vi "DBValueToDBSignal.vi"(11 "AValue":string) -> (3 "DBSignal":T1 {"Message_Type" items=["CAN", "CANFD", "J1939"]; "Mux_Type" items=["Normal", "multiplexor", "multiplexed"]; "Is_Motorola" items=["Intel", "Motorola"]; "Value_Type" items=["unsigned int", "signed int", "float", "double"]; "ID" format="%.0x"})   [LabVIEW 2014]
uses:
  Typedef/DBSignal.ctl
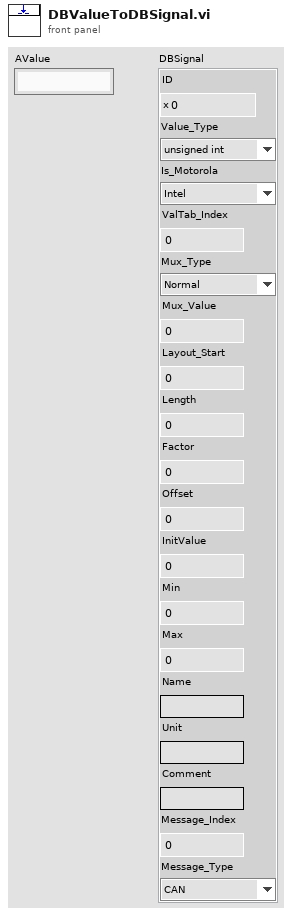
[diagram p1: front panel]
types:
  T1 = typedef "DBSignal.ctl" = cluster{"ID":i32, "Value_Type":i32, "Is_Motorola":i32, "ValTab_Index":i32, "Mux_Type":i32, "Mux_Value":dbl, "Layout_Start":i32, "Length":i32, "Factor":dbl, "Offset":dbl, "InitValue":dbl, "Min":dbl, "Max":dbl, "Name":string, "Unit":string, "Comment":string, "Message_Index":i32, "Message_Type":i32}
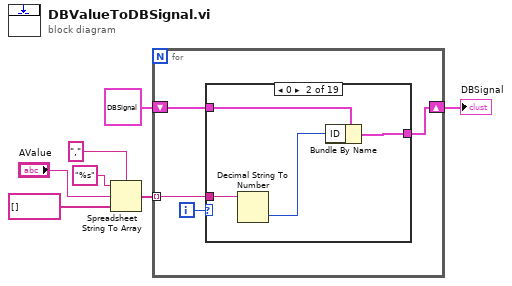
[diagram p0: block diagram]
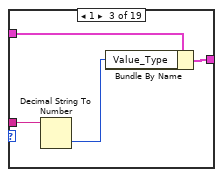
[diagram p3: hidden frame]
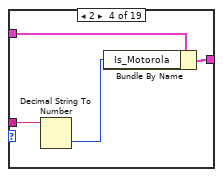
[diagram p4: hidden frame]
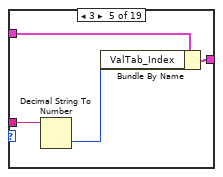
[diagram p5: hidden frame]
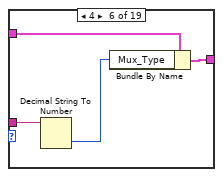
[diagram p6: hidden frame]
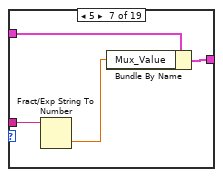
[diagram p7: hidden frame]
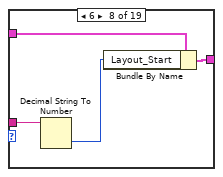
[diagram p8: hidden frame]
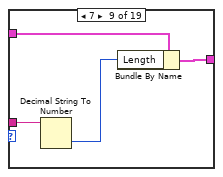
[diagram p9: hidden frame]
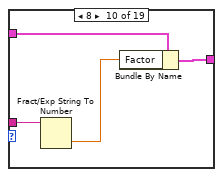
[diagram p10: hidden frame]
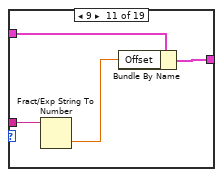
[diagram p11: hidden frame]
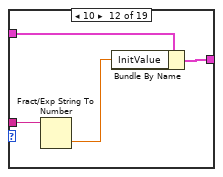
[diagram p12: hidden frame]
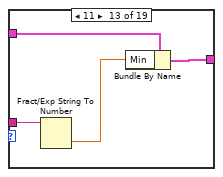
[diagram p13: hidden frame]
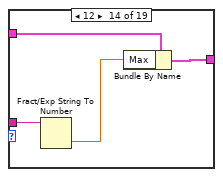
[diagram p14: hidden frame]
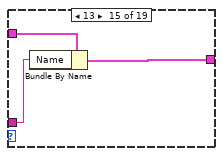
[diagram p15: hidden frame]
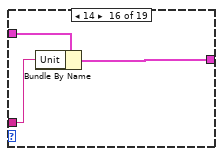
[diagram p16: hidden frame]
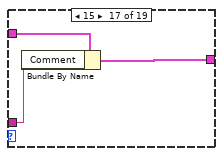
[diagram p17: hidden frame]
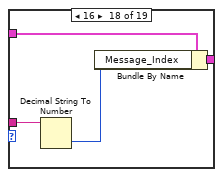
[diagram p18: hidden frame]
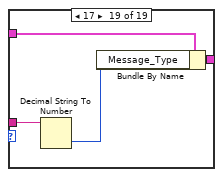
[diagram p19: hidden frame]
diagram:
  n1 = Spreadsheet String To Array(delimiter (Tab)=",", format string="%s", spreadsheet string="AValue", array type (2D Dbl)=string[] []) -> (array=w4:string[])
  n2 = for {
    tunnel: w4 -> [w9] mode=indexing
    shift-right: [w8] -> w6
    shift-left: T1 {"ID"=0, "Value_Type"=0, "Is_Motorola"=0, "ValTab_Index"=0, "Mux_Type"=0, "Mux_Value"=0.0, "Layout_Start"=0, "Length"=0, "Factor"=0.0, "Offset"=0.0, "InitValue"=0.0, "Min"=0.0, "Max"=0.0, "Name"="", "Unit"="", "Comment"="", "Message_Index"=0, "Message_Type"=0} ("DBSignal") -> [w10]
    i -> [w11]
    n3 = case shown="0" w11 {
      tunnel: w10 -> [w12 w16 w20 w24 w28 w32 w36 w40 w44 w48 w52 w56 w60 w64 w67 w70 w73 w77 w81]
      tunnel: w9 -> [_ w15 w19 w23 w27 w31 w35 w39 w43 w47 w51 w55 w59 w63 w65 w68 w71 w75 w79]
      tunnel: [w12 w13 w17 w21 w25 w29 w33 w37 w41 w45 w49 w53 w57 w61 w66 w69 w72 w76 w80] -> w8
      frame Default {
      }
      frame 0 {
        n4 = Decimal String To Number(string=w15) -> (number=w14:i32)  [unwired: 2 in, 1 out]
        n5 = Bundle By Name(cluster=w16, "ID"=w14) -> (w13:T1)
      }
      frame 1 {
        n6 = Decimal String To Number(string=w19) -> (number=w18:i32)  [unwired: 2 in, 1 out]
        n7 = Bundle By Name(cluster=w20, "Value_Type"=w18) -> (w17:T1)
      }
      frame 2 {
        n8 = Decimal String To Number(string=w23) -> (number=w22:i32)  [unwired: 2 in, 1 out]
        n9 = Bundle By Name(cluster=w24, "Is_Motorola"=w22) -> (w21:T1)
      }
      frame 3 {
        n10 = Decimal String To Number(string=w27) -> (number=w26:i32)  [unwired: 2 in, 1 out]
        n11 = Bundle By Name(cluster=w28, "ValTab_Index"=w26) -> (w25:T1)
      }
      frame 4 {
        n12 = Decimal String To Number(string=w31) -> (number=w30:i32)  [unwired: 2 in, 1 out]
        n13 = Bundle By Name(cluster=w32, "Mux_Type"=w30) -> (w29:T1)
      }
      frame 5 {
        n14 = Fract/Exp String To Number(string=w35) -> (number=w34:dbl)  [unwired: 3 in, 1 out]
        n15 = Bundle By Name(cluster=w36, "Mux_Value"=w34) -> (w33:T1)
      }
      frame 6 {
        n16 = Decimal String To Number(string=w39) -> (number=w38:i32)  [unwired: 2 in, 1 out]
        n17 = Bundle By Name(cluster=w40, "Layout_Start"=w38) -> (w37:T1)
      }
      frame 7 {
        n18 = Decimal String To Number(string=w43) -> (number=w42:i32)  [unwired: 2 in, 1 out]
        n19 = Bundle By Name(cluster=w44, "Length"=w42) -> (w41:T1)
      }
      frame 8 {
        n20 = Fract/Exp String To Number(string=w47) -> (number=w46:dbl)  [unwired: 3 in, 1 out]
        n21 = Bundle By Name(cluster=w48, "Factor"=w46) -> (w45:T1)
      }
      frame 9 {
        n22 = Fract/Exp String To Number(string=w51) -> (number=w50:dbl)  [unwired: 3 in, 1 out]
        n23 = Bundle By Name(cluster=w52, "Offset"=w50) -> (w49:T1)
      }
      frame 10 {
        n24 = Fract/Exp String To Number(string=w55) -> (number=w54:dbl)  [unwired: 3 in, 1 out]
        n25 = Bundle By Name(cluster=w56, "InitValue"=w54) -> (w53:T1)
      }
      frame 11 {
        n26 = Fract/Exp String To Number(string=w59) -> (number=w58:dbl)  [unwired: 3 in, 1 out]
        n27 = Bundle By Name(cluster=w60, "Min"=w58) -> (w57:T1)
      }
      frame 12 {
        n28 = Fract/Exp String To Number(string=w63) -> (number=w62:dbl)  [unwired: 3 in, 1 out]
        n29 = Bundle By Name(cluster=w64, "Max"=w62) -> (w61:T1)
      }
      frame 13 {
        n30 = Bundle By Name(cluster=w67, "Name"=w65) -> (w66:T1)
      }
      frame 14 {
        n31 = Bundle By Name(cluster=w70, "Unit"=w68) -> (w69:T1)
      }
      frame 15 {
        n32 = Bundle By Name(cluster=w73, "Comment"=w71) -> (w72:T1)
      }
      frame 16 {
        n33 = Decimal String To Number(string=w75) -> (number=w74:i32)  [unwired: 2 in, 1 out]
        n34 = Bundle By Name(cluster=w77, "Message_Index"=w74) -> (w76:T1)
      }
      frame 17 {
        n35 = Decimal String To Number(string=w79) -> (number=w78:i32)  [unwired: 2 in, 1 out]
        n36 = Bundle By Name(cluster=w81, "Message_Type"=w78) -> (w80:T1)
      }
    }
  }
  "DBSignal" <- w6
